vi "Peaks select ( SubVI).vi"(0 "Locations":dbl[](array[numeric]), 1 "Amplitude":dbl[](array[numeric]), 4 "No of peaks Required":i32, 5 "Min seperation B/W peaks":dbl) -> (6 "Locations":dbl[](array[numeric]), 7 "Amplitude":dbl[](array[numeric]), 9 "No of peaks found":i32)   [LabVIEW 2017]
panel:
  out "No of iterations":i32
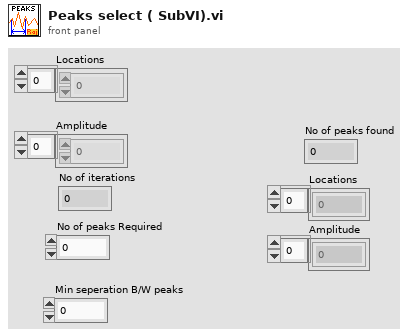
[diagram p1: front panel]
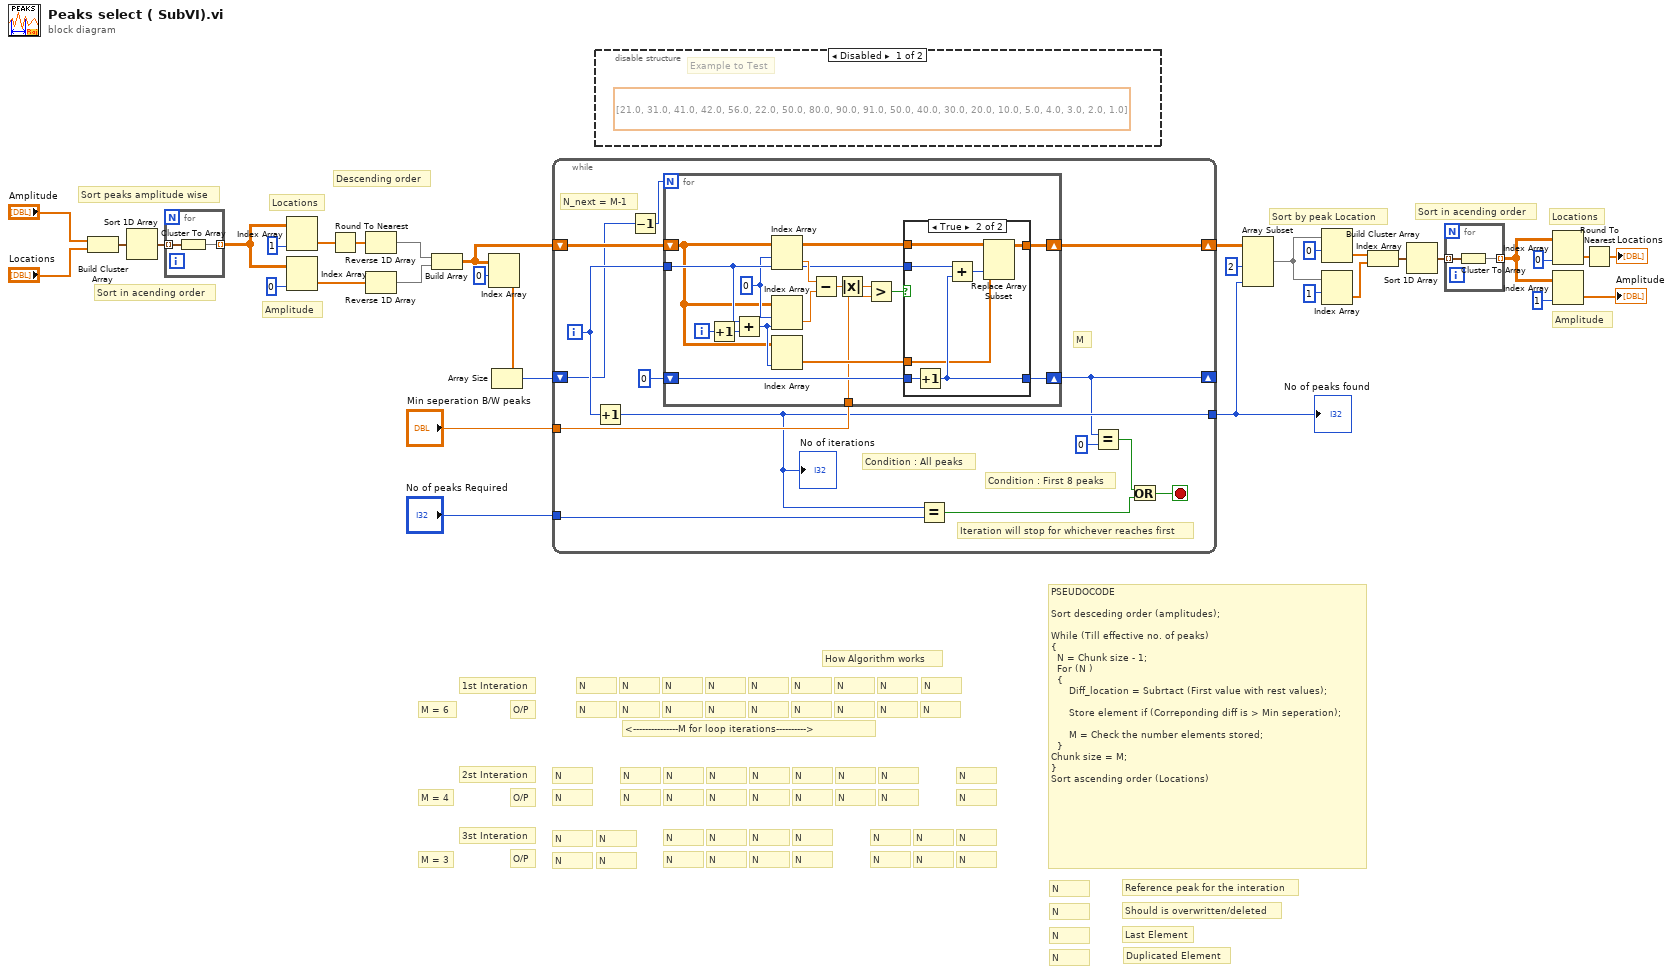
[diagram p0: block diagram]
diagram:
  # "Descending order"
  # "Sort in acending order"
  # "Locations"
  # "Amplitude"
  # "Sort peaks amplitude wise"
  # "Sort in acending order"
  # "Locations"
  # "Amplitude"
  # "Sort by peak Location"
  # "PSEUDOCODE\n\nSort desceding order (amplitudes);\n\nWhile (Till effective no. of peaks)\n{\n  N = Chunk size - 1;\n  For (N )\n  {\n      Diff_location = Subrtact (First value with rest values);\n\n      Store element if (Correponding diff is > Min seperation);\n\n      M = Check the number elements stored;\n  }\nChunk size = M;\n}\nSort ascending order (Locations)"
  # "M = 3"
  # "N"
  # "N"
  # "N"
  # "N"
  # "N"
  # "N"
  # "N"
  # "N"
  # "N"
  # "N"
  # "M = 4"
  # "M = 6"
  # "<---------------M for loop iterations---------->"
  # "N"
  # "N"
  # "N"
  # "N"
  # "N"
  # "N"
  # "N"
  # "N"
  # "N"
  # "N"
  # "N"
  # "N"
  # "O/P"
  # "3st Interation"
  # "N"
  # "N"
  # "N"
  # "N"
  # "N"
  # "N"
  # "N"
  # "N"
  # "N"
  # "Duplicated Element"
  # "N"
  # "O/P"
  # "2st Interation"
  # "O/P"
  # "N"
  # "N"
  # "N"
  # "N"
  # "N"
  # "N"
  # "N"
  # "N"
  # "N"
  # "Reference peak for the interation"
  # "N"
  # "N"
  # "N"
  # "N"
  # "N"
  # "N"
  # "N"
  # "N"
  # "N"
  # "N"
  # "1st Interation"
  # "Last Element"
  # "N"
  # "Should is overwritten/deleted"
  # "N"
  # "How Algorithm works"
  # "N"
  # "N"
  # "N"
  # "N"
  # "N"
  # "N"
  # "N"
  # "N"
  # "N"
  n1 = Build Cluster Array ("Index & Bundle Cluster Array")("Amplitude", "Locations") -> (w3:cluster{dbl, dbl}[])
  n2 = Sort 1D Array(array=w3) -> (sorted array=w4:cluster{dbl, dbl}[])
  n3 = for {
    tunnel: w4 -> [w36] mode=indexing
    tunnel: [w35] -> w9 mode=indexing
    n4 = Cluster To Array(cluster=w36) -> (array=w35:dbl[])
  }
  n5 = Index Array(array=w9, index (col)=1) -> (element=w10:dbl[])  [unwired: 1 in]
  n6 = Index Array(array=w9, index (col)=0) -> (element=w12:dbl[])  [unwired: 1 in]
  n7 = Round To Nearest(number=w10) -> (nearest integer value=w11:dbl[])
  n8 = Reverse 1D Array(array=w11) -> (reversed array=w2:dbl[])
  n9 = Reverse 1D Array(array=w12) -> (reversed array=w1:dbl[])
  n10 = Build Array(w2, w1) -> (w13:dbl[][])
  n11 = Index Array(array=w13, index (row)=0) -> (element=w31:dbl[])  [unwired: 1 in]
  n12 = Array Size(array=w31) -> (size(s)=w29:i32)
  n13 = while {
    shift-right: [w45] -> w32
    shift-left: w13 -> [w49]
    shift-right: [w37] -> _
    shift-left: w29 -> [w46]
    tunnel: "Min seperation B/W peaks" -> [w44]
    tunnel: "No of peaks Required" -> [w42]
    tunnel: [w38] -> w27
    i -> [w48]
    stop <- w39 stop-if-true
    # "Iteration will stop for whichever reaches first"
    # "Condition : First 8 peaks"
    # "Condition : All peaks"
    # "N_next = M-1"
    # "M"
    n14 = Increment(x=w48) -> (x+1=w38:i32)
    "No of iterations" <- w38
    n15 = Decrement(x=w46) -> (x-1=w47:i32)
    n16 = for {
      N: w47 -> [_]
      tunnel: w48 -> [w57]
      shift-right: [w58] -> w37
      shift-left: 0 -> [w60]
      shift-right: [w52] -> w45
      shift-left: w49 -> [w54]
      tunnel: w44 -> [w51]
      i -> [w66]
      w56 = 0 ("disabled index (row)")
      n17 = Increment(x=w66) -> (x+1=w65:i32)
      n18 = Add(x=w57, y=w65) -> (x+y=w55:i32)
      n19 = Index Array(array=w54, index (row)=w56, index (col)=w57) -> (element=w64:dbl)
      n20 = Index Array(array=w54, index (row)=w56, index (col)=w55) -> (element=w59:dbl)
      n21 = Index Array(array=w54, index (col)=w55) -> (element=w53:dbl[])  [unwired: 1 in]
      n22 = Subtract(x=w64, y=w59) -> (x-y=w63:dbl)
      n23 = Absolute Value(x=w63) -> (abs(x)=w62:dbl)
      n24 = Greater?(x=w62, y=w51) -> (0:w61:bool)
      n25 = case shown="True" w61 {
        tunnel: w60 -> [w68 w75]
        tunnel: w54 -> [w67 w74]
        tunnel: [w68 w71] -> w58
        tunnel: [w67 w73] -> w52
        tunnel: w57 -> [_ w72]
        tunnel: w53 -> [_ w69]
        frame False {
        }
        frame True {
          n26 = Increment(x=w75) -> (x+1=w71:i32)
          n27 = Add(x=w72, y=w71) -> (x+y=w70:i32)
          n28 = Replace Array Subset(array=w74, new element=w69, index (col)=w70) -> (w73:dbl[][])  [unwired: 1 in]
        }
      }
    }
    n29 = Equal?(x=w38, y=w42) -> (x = y?=w41:bool)
    n30 = Equal?(x=w37, y=0 ("x")) -> (x = y?=w40:bool)
    n31 = Or(x=w40, y=w41) -> (x .or. y?=w39:bool)
  }
  "No of peaks found" <- w27
  n32 = disable-structure shown="Disabled" {
    frame Disabled {
      (unwired) dbl[][] [[21.0, 31.0, 41.0, 42.0, 56.0, 22.0, 50.0, 80.0, 90.0, 91.0], [50.0, 40.0, 30.0, 20.0, 10.0, 5.0, 4.0, 3.0, 2.0, 1.0]]
      # "Example to Test"
    }
    frame Enabled {
    }
  }
  n33 = Array Subset(array=w32, length (row)=2 ("dimension size"), length (col)=w27) -> (w19:dbl[][])  [unwired: 2 in]
  n34 = Index Array(array=w19, index (row)=0) -> (element=w22:dbl[])  [unwired: 1 in]
  n35 = Index Array(array=w19, index (row)=1) -> (element=w18:dbl[])  [unwired: 1 in]
  n36 = Build Cluster Array ("Index & Bundle Cluster Array")(w22, w18) -> (w17:cluster{dbl, dbl}[])
  n37 = Sort 1D Array(array=w17) -> (sorted array=w23:cluster{dbl, dbl}[])
  n38 = for {
    tunnel: w23 -> [w76] mode=indexing
    tunnel: [w77] -> w26 mode=indexing
    n39 = Cluster To Array(cluster=w76) -> (array=w77:dbl[])
  }
  n40 = Index Array(array=w26, index (col)=0) -> (element=w16:dbl[])  [unwired: 1 in]
  n41 = Index Array(array=w26, index (col)=1) -> (element=→"Amplitude":dbl[])  [unwired: 1 in]
  n42 = Round To Nearest(number=w16) -> (nearest integer value=→"Locations":dbl[])
